vi "Read Event.vi"(2 "FlexChannel":T1) -> (7 "Event Reg":refnum<event-registration>)   [LabVIEW 2020, in "Flex.lvlib"]
doc: "Creates an event registration so data that is sent through the channel can be received by an event structure. This registration can be bundled with other events to pass into the dynamic event terminal of an event structure.\n\nIncluded in the event data is a boolean, Closed, that is set to true when the channel has been cleaned up. When Closed is true, the Value will be default and invalid."
uses:
  Flex.lvlib
  ChannelOp.ctl
  Element.ctl
  ))Channel.ctl
  Event Data.ctl
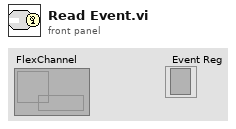
[diagram p1: front panel]
types:
  T1 = typedef "Flex.lvlib/))Channel.ctl" = refnum<queue>
  T2 = typedef "Flex.lvlib/ChannelOp.ctl" = enum16{"Get Refs", "Init", "Close", "Probe", "New Queue", "Remove Queue", "New Event"}
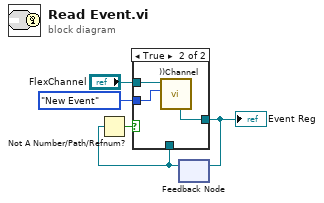
[diagram p0: block diagram]
diagram:
  n1 = feedback #1() -> (w2:refnum<event-registration>)  [unwired: 1 in]
  n2 = Not A Number/Path/Refnum?(number/path/refnum=w2) -> (NaN/Path/Refnum?=w3:bool)
  n3 = case shown="True" w3 {
    tunnel: "FlexChannel" -> [_ w9]
    tunnel: ChannelOp."New Event" ("channelOp") -> [_ w8]
    tunnel: [w6 w7] -> w1
    tunnel: w2 -> [w6 _]
    frame False {
    }
    frame True {
      n4 = call "))Channel.vi"("channelOp"=w8, "channel in"=w9) -> ("Event Reg"=w7:refnum<event-registration>)  [unwired: 5 in, 4 out]
    }
  }
  "Event Reg" <- w1
  n5 = feedback-in #1(w1) -> ()
